vi "Read Section Packet Refs.vi"(8 "error in (no error)":errorcluster, 11 "Node Ptr":T1 format="%.0x") -> (0 "error out":errorcluster, 2 "Dependent Node Refs":T1[](array[typedef]) format="%.0x", 3 "Node Ptr out":T1 format="%.0x")   [LabVIEW 2019, in "UDP-Custom-Device System Explorer.lvlib" / "Shared Section Accessors.lvlib"]
uses:
  Shared Section Accessors.lvlib
  <vilib>/NI VeriStand/Custom Device API/Custom Device Item Ref.ctl
  Shared/Constants.vi
  Shared/UDP-Custom-Device Shared.lvlib
  <vilib>/NI VeriStand/Custom Device Tools/Custom Device Utility Library/Custom Device Utility Library.lvlib
  <vilib>/NI VeriStand/Custom Device API/Custom Device API.lvlib
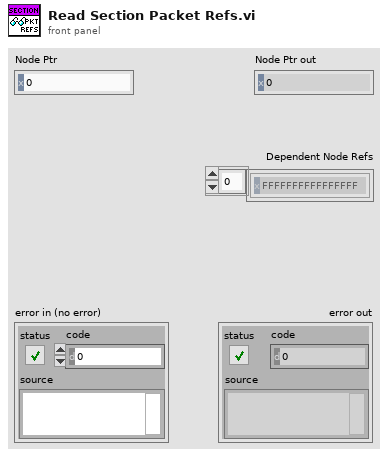
[diagram p1: front panel]
types:
  T1 = typedef "Custom Device API.lvlib/Custom Device Item Ref.ctl" = u64
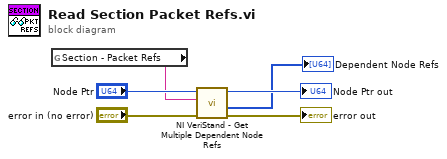
[diagram p0: block diagram]
diagram:
  n1 = global read "Constants.vi" "Section - Packet Refs"() -> (w2:string)
  n2 = call <vilib>:"NI VeriStand - Get Multiple Dependent Node Refs.vi"("error in (no error)"="error in (no error)", "Base Property Name"=w2, "Item Ref in"="Node Ptr") -> ("error out"=→"error out":errorcluster, "Dependent Node Refs"=→"Dependent Node Refs":T1[], "Item Ref out"=→"Node Ptr out":T1)  [unwired: 6 in]
